vi "AI2Degree.vi"(5 "Gear":dbl=1.0, 6 "Invert":bool, 7 "Calibrate":dbl=66.987, 11 "AIDeviceRef":T1) -> (1 "Degree":dbl)   [LabVIEW 2012]
uses:
  <vilib>/Rock Robotics/WPI/AnalogChannel/WPI_AnalogChannelDevRef.ctl
  <vilib>/Rock Robotics/SystemInterfaces/Typedef/FPGA_TypedefAnalogModule.ctl
  <vilib>/Rock Robotics/SystemInterfaces/AI/FPGA_AIChannel.ctl
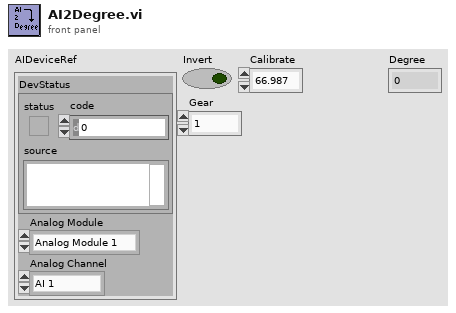
[diagram p1: front panel]
types:
  T1 = typedef "WPI_AnalogChannelDevRef.ctl" = cluster{"DevStatus":errorcluster, "Analog Module":T2, "Analog Channel":T3}
  T2 = typedef "FPGA_TypedefAnalogModule.ctl" = enum16{"Analog Module 1", "Analog Module 2"}
  T3 = typedef "FPGA_AIChannel.ctl" = enum8{"AI 1", "AI 2", "AI 3", "AI 4", "AI 5", "AI 6", "AI 7", "AI 8", "Invalid"}
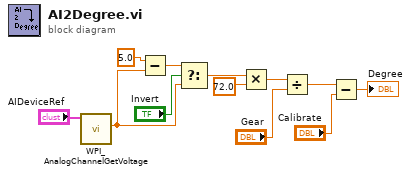
[diagram p0: block diagram]
diagram:
  n1 = call <vilib>:"WPI_AnalogChannelGetVoltage.vi"("AIDeviceRef"="AIDeviceRef") -> ("Voltage"=w8:dbl)  [unwired: 8 in, 2 out]
  n2 = Subtract(x=5.0, y=w8) -> (x-y=w7:dbl)
  n3 = Select(t=w7, s="Invert", f=w8) -> (s? t:f=w6:dbl)
  n4 = Multiply(x=w6, y=72.0) -> (x*y=w5:dbl)
  n5 = Divide(x=w5, y="Gear") -> (x/y=w3:dbl)
  n6 = Subtract(x=w3, y="Calibrate") -> (x-y=→"Degree":dbl)
